vi "Climber Debug.vi"   [LabVIEW 2012]
uses:
  <vilib>/Rock Robotics/WPI/Solenoid/WPI_SolenoidValue.ctl
  <vilib>/Rock Robotics/WPI/Relay/WPI_RelayValue.ctl
  Robot Global Data.vi
  <vilib>/Rock Robotics/WPI/Solenoid/WPI_SolenoidSetEnum.vi
  <vilib>/Rock Robotics/WPI/RobotDrive/WPI_RobotDriveGetSetRefNum.vi
types:
  T1 = typedef "WPI_JoystickButtonState.ctl" = cluster{"Button 1":bool, "Button 2":bool, "Button 3":bool, "Button 4":bool, "Button 5":bool, "Button 6":bool, "Button 7":bool, "Button 8":bool, "Button 9":bool, "Button 10":bool, "Button 11":bool, "Button 12":bool}
  T2 = typedef "WPI_RelayValue.ctl" = enum16{"Off", "On", "Forward", "Reverse"}
  T3 = typedef "WPI_RelayDevRef.ctl" = cluster{"DevStatus":errorcluster, "Relay Channel":T4, "Digital Module":T5, "Relay Direction":T6}
  T4 = typedef "FPGA_DIORelayChannel.ctl" = enum8{"Relay 1", "Relay 2", "Relay 3", "Relay 4", "Relay 5", "Relay 6", "Relay 7", "Relay 8", "Invalid"}
  T5 = typedef "FPGA_TypedefDigitalModule.ctl" = enum16{"Digital Module 1", "Digital Module 2"}
  T6 = typedef "WPI_RelayDirection.ctl" = enum16{"Both directions", "Forward only", "Reverse only"}
  T7 = typedef "WPI_RobotDriveDevRef.ctl" = cluster{"DevStatus":errorcluster, "Motors[]":T8[], "Square Inputs":bool, "Max Output":dbl, "Isochronous":bool}
  T8 = typedef "WPI_MotorControlDeviceRef.ctl" = cluster{"DeviceStatus":errorcluster, "Type":enum16{"PWM", "CAN"}, "PWM":cluster{"Digital Module":T5, "PWM Channel":T9, "DeadBand":T10}, "CAN":cluster{"Device Number":u8, "Control Mode":T11, "Semaphore":T12, "Max Vout":dbl}, "Invert":bool, "TransformRef":T13, "InvTransformRef":T13}
  T9 = typedef "FPGA_DIOPWMChannel.ctl" = enum8{"PWM 1", "PWM 2", "PWM 3", "PWM 4", "PWM 5", "PWM 6", "PWM 7", "PWM 8", "PWM 9", "PWM 10", "Invalid"}
  T10 = typedef "WPI_PWMDeadband.ctl" = cluster{"Name":string, "maxPositivePwm":i32, "minPositivePwm":i32, "centerPwm":i32, "maxNegativePwm":i32, "minNegativePwm":i32, "angularRange":u16}
  T11 = typedef "WPI_CANJaguar_ControlMode.ctl" = enum8{"Percent VBus", "Current", "Speed", "Position", "Voltage"}
  T12 = typedef "Semaphore RefNum" = refnum<k1>
  T13 = typedef "WPI_PWMTransform_ConPane.ctl" = refnum<vi>
  T14 = typedef "WPI_SolenoidValue.ctl" = enum16{"Off", "On", "Forward", "Reverse"}
  T15 = typedef "WPI_SolenoidDevRef.ctl" = cluster{"DevStatus":errorcluster, "Solenoid Module":T16, "Forward Solenoid Channel":T17, "Reverse Solenoid Channel":T17}
  T16 = typedef "FPGA_TypedefSolenoidModule.ctl" = enum16{"Solenoid Module 1", "Solenoid Module 2"}
  T17 = typedef "WPI_SolenoidChannel.ctl" = enum8{"Solenoid 1", "Solenoid 2", "Solenoid 3", "Solenoid 4", "Solenoid 5", "Solenoid 6", "Solenoid 7", "Solenoid 8", "Invalid"}
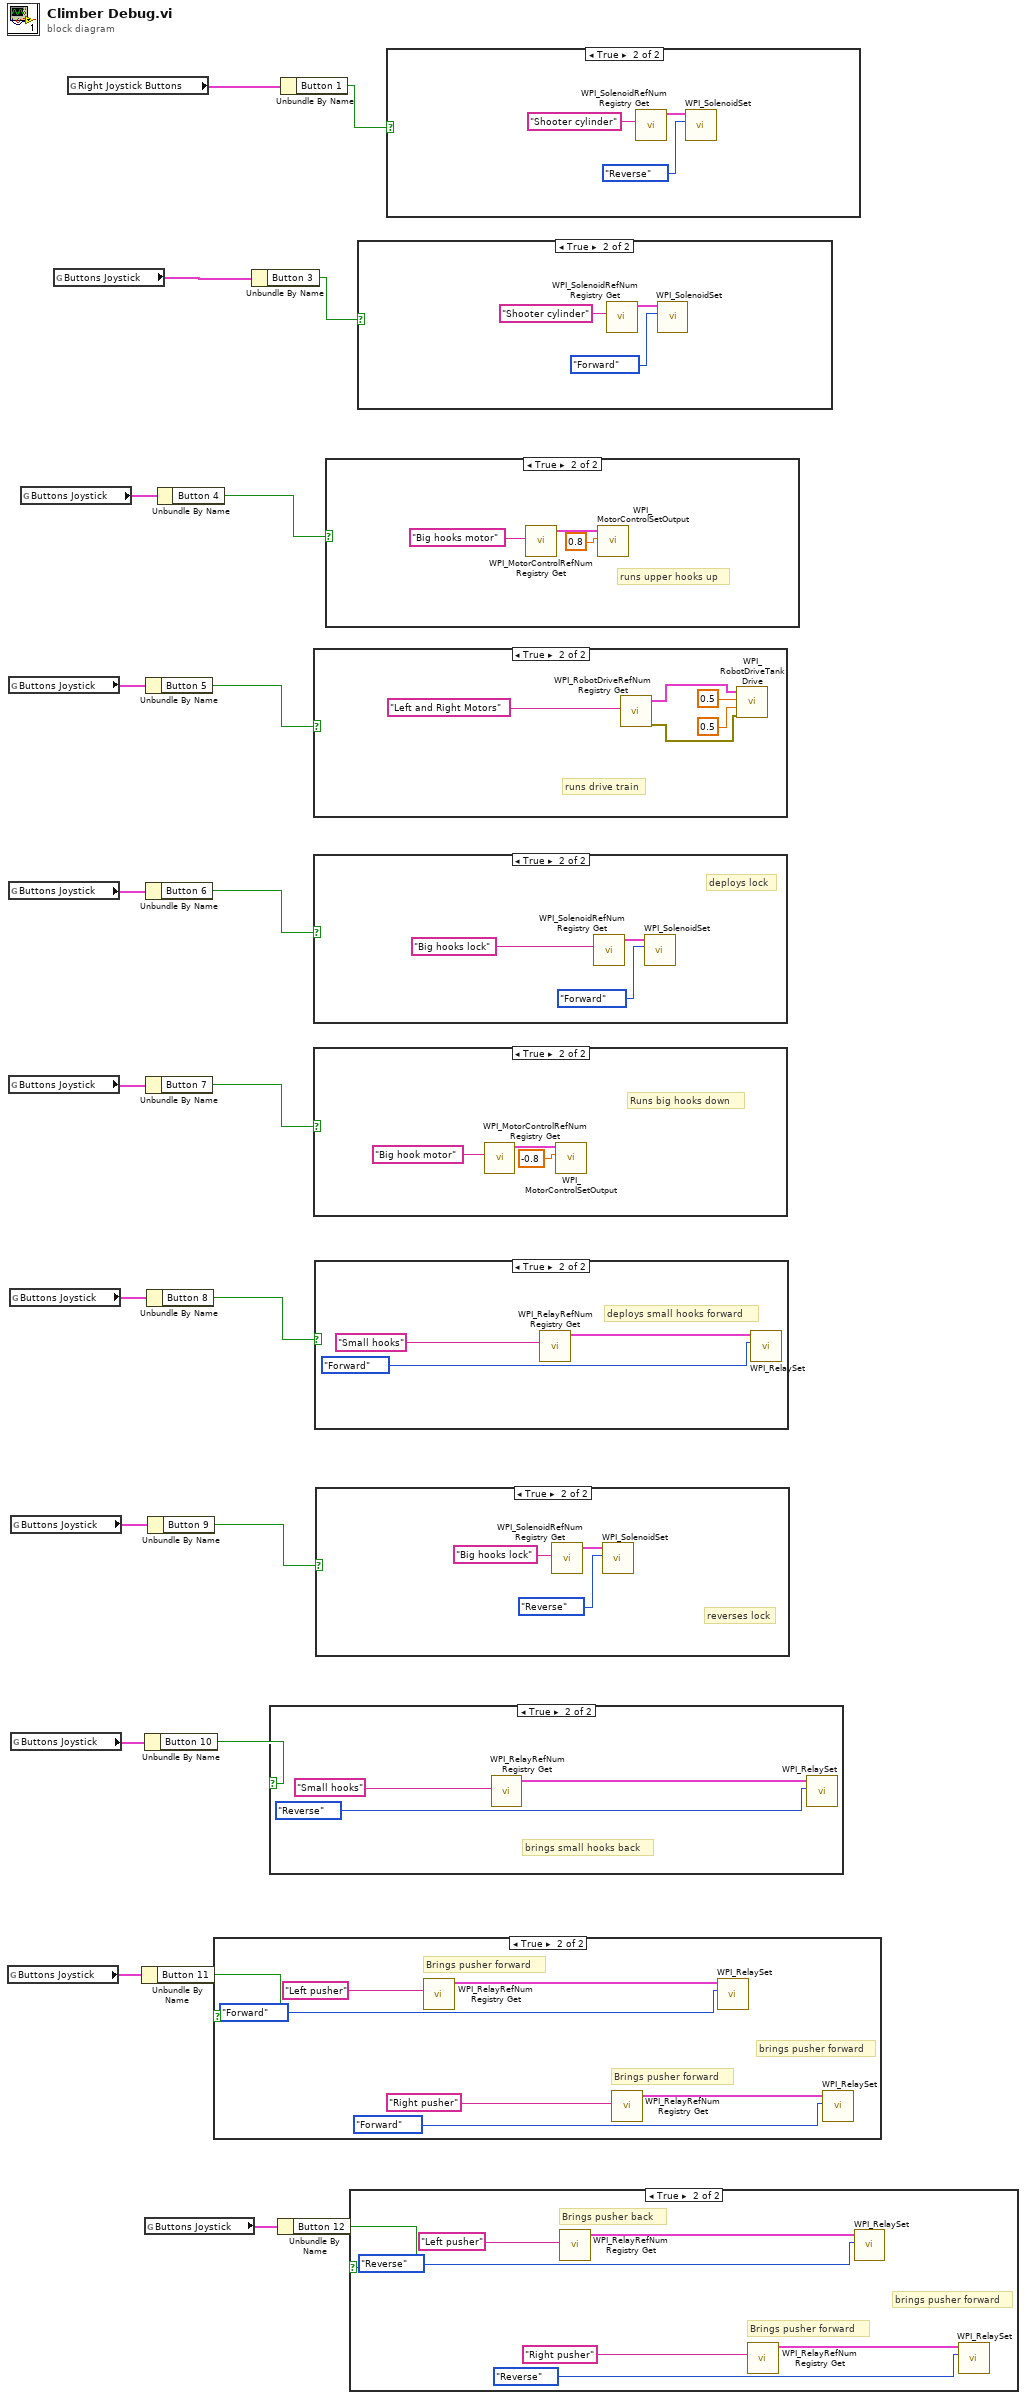
[diagram p0: block diagram]
diagram:
  n1 = global read "Robot Global Data.vi" "Buttons Joystick"() -> (w6:T1)
  n2 = global read "Robot Global Data.vi" "Buttons Joystick"() -> (w18:T1)
  n3 = global read "Robot Global Data.vi" "Buttons Joystick"() -> (w16:T1)
  n4 = global read "Robot Global Data.vi" "Buttons Joystick"() -> (w14:T1)
  n5 = global read "Robot Global Data.vi" "Buttons Joystick"() -> (w12:T1)
  n6 = global read "Robot Global Data.vi" "Buttons Joystick"() -> (w10:T1)
  n7 = global read "Robot Global Data.vi" "Buttons Joystick"() -> (w8:T1)
  n8 = global read "Robot Global Data.vi" "Buttons Joystick"() -> (w20:T1)
  n9 = global read "Robot Global Data.vi" "Buttons Joystick"() -> (w22:T1)
  n10 = global read "Robot Global Data.vi" "Right Joystick Buttons"() -> (w2:T1)
  n11 = Unbundle By Name(w6) -> ("Button 11"=w5:bool)
  n12 = Unbundle By Name(w8) -> ("Button 10"=w7:bool)
  n13 = global read "Robot Global Data.vi" "Buttons Joystick"() -> (w4:T1)
  n14 = Unbundle By Name(w18) -> ("Button 5"=w17:bool)
  n15 = Unbundle By Name(w16) -> ("Button 6"=w15:bool)
  n16 = Unbundle By Name(w14) -> ("Button 7"=w13:bool)
  n17 = Unbundle By Name(w12) -> ("Button 8"=w11:bool)
  n18 = Unbundle By Name(w10) -> ("Button 9"=w9:bool)
  n19 = Unbundle By Name(w20) -> ("Button 4"=w19:bool)
  n20 = case shown="True" w5 {
    frame False {
    }
    frame True {
      # "brings pusher forward"
      # "Brings pusher forward"
      # "Brings pusher forward"
      n21 = call <vilib>:"WPI_RelayRefNum Registry Get.vi"("refnum name"="Left pusher") -> ("RelayDevRef"=w28:T3)  [unwired: 9 in, 1 out]
      n22 = call <vilib>:"WPI_RelayRefNum Registry Get.vi"("refnum name"="Right pusher") -> ("RelayDevRef"=w25:T3)  [unwired: 9 in, 1 out]
      n23 = call <vilib>:"WPI_RelaySet.vi"("RelayValue"=WPI_RelayValue."Forward", "RelayDevRef"=w28) -> ()  [unwired: 8 in, 2 out]
      n24 = call <vilib>:"WPI_RelaySet.vi"("RelayValue"=WPI_RelayValue."Forward", "RelayDevRef"=w25) -> ()  [unwired: 8 in, 2 out]
    }
  }
  n25 = Unbundle By Name(w22) -> ("Button 3"=w21:bool)
  n26 = case shown="True" w7 {
    frame False {
    }
    frame True {
      # "brings small hooks back"
      n27 = call <vilib>:"WPI_RelayRefNum Registry Get.vi"("refnum name"="Small hooks") -> ("RelayDevRef"=w31:T3)  [unwired: 9 in, 1 out]
      n28 = call <vilib>:"WPI_RelaySet.vi"("RelayValue"=WPI_RelayValue."Reverse", "RelayDevRef"=w31) -> ()  [unwired: 8 in, 2 out]
    }
  }
  n29 = Unbundle By Name(w4) -> ("Button 12"=w3:bool)
  n30 = Unbundle By Name(w2) -> ("Button 1"=w1:bool)
  n31 = case shown="True" w17 {
    frame False {
    }
    frame True {
      # "runs drive train"
      n32 = call <vilib>:"WPI_RobotDriveRefNum Registry Get.vi"("refnum name"="Left and Right Motors") -> ("error out"=w36:errorcluster, "RobotDriveDevRef"=w35:T7)  [unwired: 1 in, 8 out]
      n33 = call <vilib>:"WPI_RobotDriveTankDrive.vi"("error in (no error)"=w36, "Right axis value"=0.5, "Left axis value"=0.5, "RobotDriveDevRef"=w35) -> ()  [unwired: 5 in, 3 out]
    }
  }
  n34 = case shown="True" w15 {
    frame False {
    }
    frame True {
      # "deploys lock"
      n35 = call <vilib>:"WPI_SolenoidRefNum Registry Get.vi"("refnum name"="Big hooks lock") -> ("SolenoidDevRef"=w38:T15)  [unwired: 9 in, 1 out]
      n36 = call-poly <vilib>:"WPI_SolenoidSet.vi"("Value"=WPI_SolenoidValue."Forward", "SolenoidDevRef"=w38) -> ()  [unwired: 8 in, 2 out]
    }
  }
  n37 = case shown="True" w13 {
    frame False {
    }
    frame True {
      # "Runs big hooks down"
      n38 = call <vilib>:"WPI_MotorControlRefNum Registry Get.vi"("refnum name"="Big hook motor") -> ("MotorControlDevRef"=w42:T8)  [unwired: 9 in, 1 out]
      n39 = call <vilib>:"WPI_MotorControlSetOutput.vi"("Output"=-0.8, "MotorControlDevRef"=w42) -> ()  [unwired: 7 in, 3 out]
    }
  }
  n40 = case shown="True" w11 {
    frame False {
    }
    frame True {
      # "deploys small hooks forward"
      n41 = call <vilib>:"WPI_RelayRefNum Registry Get.vi"("refnum name"="Small hooks") -> ("RelayDevRef"=w45:T3)  [unwired: 9 in, 1 out]
      n42 = call <vilib>:"WPI_RelaySet.vi"("RelayValue"=WPI_RelayValue."Forward", "RelayDevRef"=w45) -> ()  [unwired: 8 in, 2 out]
    }
  }
  n43 = case shown="True" w9 {
    frame False {
    }
    frame True {
      # "reverses lock"
      n44 = call <vilib>:"WPI_SolenoidRefNum Registry Get.vi"("refnum name"="Big hooks lock") -> ("SolenoidDevRef"=w47:T15)  [unwired: 9 in, 1 out]
      n45 = call-poly <vilib>:"WPI_SolenoidSet.vi"("Value"=WPI_SolenoidValue."Reverse", "SolenoidDevRef"=w47) -> ()  [unwired: 8 in, 2 out]
    }
  }
  n46 = case shown="True" w19 {
    frame False {
    }
    frame True {
      # "runs upper hooks up"
      n47 = call <vilib>:"WPI_MotorControlRefNum Registry Get.vi"("refnum name"="Big hooks motor") -> ("MotorControlDevRef"=w49:T8)  [unwired: 9 in, 1 out]
      n48 = call <vilib>:"WPI_MotorControlSetOutput.vi"("Output"=0.8, "MotorControlDevRef"=w49) -> ()  [unwired: 7 in, 3 out]
    }
  }
  n49 = case shown="True" w3 {
    frame False {
    }
    frame True {
      # "brings pusher forward"
      # "Brings pusher forward"
      # "Brings pusher back"
      n50 = call <vilib>:"WPI_RelayRefNum Registry Get.vi"("refnum name"="Left pusher") -> ("RelayDevRef"=w57:T3)  [unwired: 9 in, 1 out]
      n51 = call <vilib>:"WPI_RelayRefNum Registry Get.vi"("refnum name"="Right pusher") -> ("RelayDevRef"=w54:T3)  [unwired: 9 in, 1 out]
      n52 = call <vilib>:"WPI_RelaySet.vi"("RelayValue"=WPI_RelayValue."Reverse", "RelayDevRef"=w57) -> ()  [unwired: 8 in, 2 out]
      n53 = call <vilib>:"WPI_RelaySet.vi"("RelayValue"=WPI_RelayValue."Reverse", "RelayDevRef"=w54) -> ()  [unwired: 8 in, 2 out]
    }
  }
  n54 = case shown="True" w21 {
    frame False {
    }
    frame True {
      n55 = call <vilib>:"WPI_SolenoidRefNum Registry Get.vi"("refnum name"="Shooter cylinder") -> ("SolenoidDevRef"=w59:T15)  [unwired: 9 in, 1 out]
      n56 = call-poly <vilib>:"WPI_SolenoidSet.vi"("Value"=WPI_SolenoidValue."Forward", "SolenoidDevRef"=w59) -> ()  [unwired: 8 in, 2 out]
    }
  }
  n57 = case shown="True" w1 {
    frame False {
    }
    frame True {
      n58 = call <vilib>:"WPI_SolenoidRefNum Registry Get.vi"("refnum name"="Shooter cylinder") -> ("SolenoidDevRef"=w62:T15)  [unwired: 9 in, 1 out]
      n59 = call-poly <vilib>:"WPI_SolenoidSet.vi"("Value"=WPI_SolenoidValue."Reverse", "SolenoidDevRef"=w62) -> ()  [unwired: 8 in, 2 out]
    }
  }
